vi "Read RTU Data.vi"(8 "error in (no error)":errorcluster, 10 "function code":u8=1 format="%x", 11 "MODBUS in":refnum<class "Modbus.lvclass">) -> (0 "error out":errorcluster, 2 "data":string, 3 "MODBUS Out":refnum<class "Modbus.lvclass">)   [LabVIEW 2020, in "Library Instrument & Equipement.lvlib" / "Library Relay_Board.lvlib" / "Modbus.lvclass"]
doc: "Reads RTU frame data. Override this VI for not implemented and user-defined Modbus function code(s)."
uses:
  Modbus.lvclass
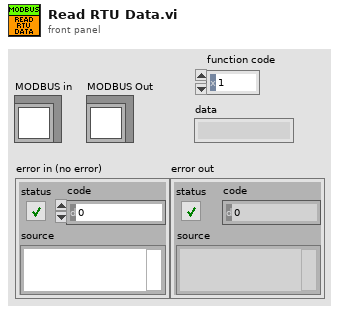
[diagram p1: front panel]
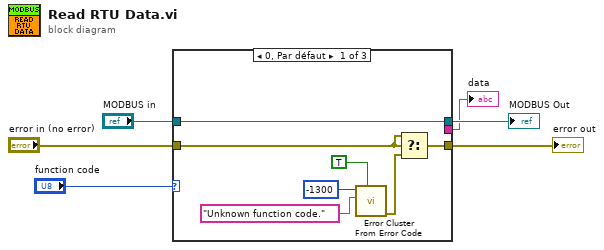
[diagram p0: block diagram]
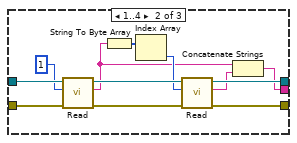
[diagram p2: hidden frame]
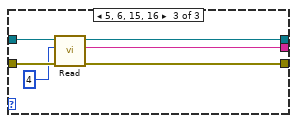
[diagram p3: hidden frame]
diagram:
  n1 = case shown="0, Par défaut" "function code" {
    tunnel: "error in (no error)" -> [w8 w25 w30]
    tunnel: [w9 w20 w27] -> w2
    tunnel: "MODBUS in" -> [w10 w24 w31]
    tunnel: [w10 w21 w28] -> w4
    tunnel: [_ w14 w26] -> w3
    frame 0, Default {
      n2 = call <vilib>:"Error Cluster From Error Code.vi"("show call chain? (False)"=TRUE, "error message (\"\")"="Unknown function code." ("format string"), "error code (0)"=-1300) -> ("error out"=w7:errorcluster)  [unwired: 6 in]
      n3 = Select(t=w8, s=w8, f=w7) -> (s? t:f=w9:errorcluster)
    }
    frame 1..4 {
      n4 = call "Read.vi"("error in (no error)"=w25, "byte count"=u32 1, "MODBUS in"=w24) -> ("error out"=w17:errorcluster, "read buffer"=w16:string, "MODBUS Out"=w22:refnum<class "Modbus.lvclass">)  [unwired: 6 in]
      n5 = String To Byte Array(string=w16) -> (unsigned byte array=w19:u8[])
      n6 = Index Array(array=w19) -> (element=w18:u8)  [unwired: 1 in]
      n7 = call "Read.vi"("error in (no error)"=w17, "byte count"=w18, "MODBUS in"=w22) -> ("error out"=w20:errorcluster, "read buffer"=w15:string, "MODBUS Out"=w21:refnum<class "Modbus.lvclass">)  [unwired: 6 in]
      n8 = Concatenate Strings(w16, w15) -> (w14:string)
    }
    frame 5, 6, 15, 16 {
      n9 = call "Read.vi"("error in (no error)"=w30, "byte count"=u32 4, "MODBUS in"=w31) -> ("error out"=w27:errorcluster, "read buffer"=w26:string, "MODBUS Out"=w28:refnum<class "Modbus.lvclass">)  [unwired: 6 in]
    }
  }
  "MODBUS Out" <- w4
  "data" <- w3
  "error out" <- w2
